vi "Remove invalid folder characters.vi"(8 "error in (no error)":errorcluster, 11 "String in":string) -> (0 "error out":errorcluster, 3 "String out":string)   [LabVIEW 2016]
doc: "This VI searches for the characters \\/:*?\"<>| in the input string. If any are present, they are removed.The resulting string is then generated."
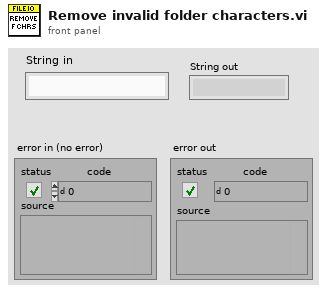
[diagram p1: front panel]
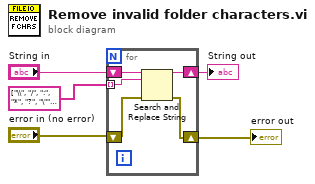
[diagram p0: block diagram]
diagram:
  n1 = for {
    tunnel: string[] ["\\", "/", ":", "*", "?", "\"", "<", ">", "|"] -> [w9] mode=indexing
    shift-right: [w8] -> w1
    shift-left: "String in" -> [w10]
    shift-right: [w6] -> w2
    shift-left: "error in (no error)" -> [w7]
    n2 = Search and Replace String(input string=w10, search string=w9, error in=w7) -> (result string=w8:string, error out=w6:errorcluster)  [unwired: 5 in, 2 out]
  }
  "error out" <- w2
  "String out" <- w1
